vi "getCursorPosition.vi"(6 "Cursos id":i32, 7 "reference":refnum<vi>) -> (0 "Position.Y":dbl, 1 "Position.X":dbl, 2 "error out":errorcluster, 3 "reference out":refnum<vi>)   [LabVIEW 2014]
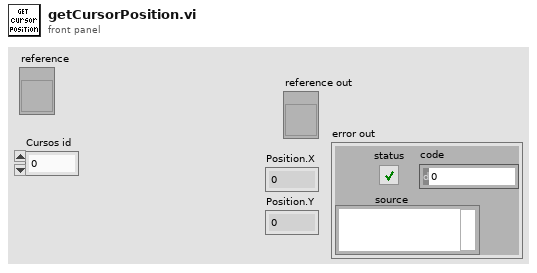
[diagram p1: front panel]
types:
  T1 = typedef "LVCursorListTypeDef.ctl" = cluster{"Name":string, "Color":u32, "Style":u8, "Point Style":u8, "Name Visible":bool, "Allow Drag":bool, "Cursor Mode":u32, "Plot":i32, "Index":i32, "Position":cluster{"X":dbl, "Y":dbl}, "X Scale":u32, "Y Scale":u32, "Watch Plots":i32[], "Watch All Plots":bool, "Plot Area":i32, "Label Offset":cluster{"X":dbl, "Y":dbl}}[]
  T2 = cluster{"Name":string, "Color":u32, "Style":u8, "Point Style":u8, "Name Visible":bool, "Allow Drag":bool, "Cursor Mode":u32, "Plot":i32, "Index":i32, "Position":cluster{"X":dbl, "Y":dbl}, "X Scale":u32, "Y Scale":u32, "Watch Plots":i32[], "Watch All Plots":bool, "Plot Area":i32, "Label Offset":cluster{"X":dbl, "Y":dbl}}
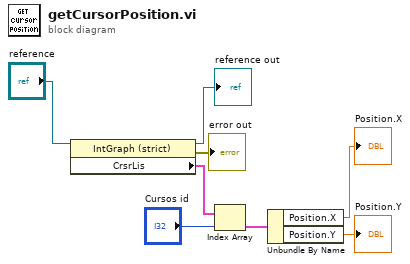
[diagram p0: block diagram]
diagram:
  n1 = property on="Property Node" class="IntGraph (strict)"(reference="reference") -> (reference out=→"reference out":refnum<vi>, error out=→"error out":errorcluster, "CrsrLis"=w7:T1)  [unwired: 1 in]
  n2 = Index Array(array=w7, index="Cursos id") -> (element=w6:T2)
  n3 = Unbundle By Name(w6) -> ("Position.X"=→"Position.X":dbl, "Position.Y"=→"Position.Y":dbl)
